vi "Element Init.vi"(7 "VolatusAPI":refnum<class "VolatusAPI.lvclass">, 8 "error in (no error)":errorcluster, 10 "JSON":string, 11 "HtmlButtonControl in":refnum<class "HttpButtonControl.lvclass">) -> (0 "error out":errorcluster, 3 "HtmlButtonControl out":refnum<class "HttpButtonControl.lvclass">)   [LabVIEW 2020, in "VolatusGUIElements.lvlib" / "HttpButtonControl.lvclass"]
uses:
  HttpButtonControl.lvclass
  C:/dev/lv20CE/relink/lv-volatus/VolatusGUI/GUI Element/GUI Element.lvclass
  Volatus/VolatusAPI/VolatusAPI.lvclass
  JSON.ctl
  Method.ctl
  VolatusGUI/GUI Element/GUI Element.lvclass/GUI Element.ctl
  HttpButtonControl.lvclass/HttpButtonControl.ctl
  af0a34e3-17dd-43c9-97df-e95964bc46e3.vi
  <vilib>/JDP Science/JSONtext/JSON text to Variant.vi
  <vilib>/JDP Science/JSONtext/LVClass Serializer/JSONtext LVClass Serializer.lvclass
  VolatusGUI/GUI Element/GUI Element.lvclass
  C:/dev/lv20CE/relink/lv-volatus/VolatusGUIElements/HttpButtonControl/HttpButtonControl.lvclass
  C:/dev/lv20CE/relink/lv-volatus/VolatusGUI/OnValueChangeHandler/OnValueChangeHandler.lvclass
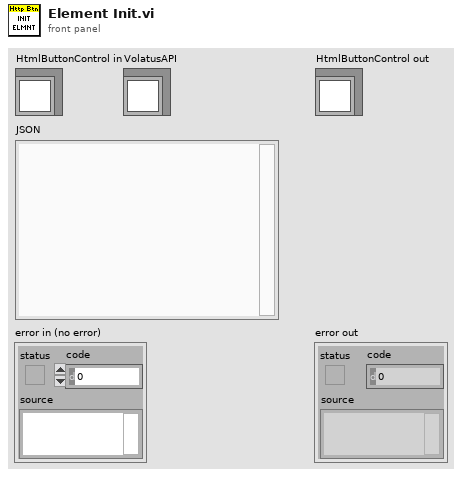
[diagram p1: front panel]
types:
  T1 = typedef "VolatusGUIElements.lvlib/HttpButtonControl.lvclass/Method.ctl" = enum16{"Get", "Post"}
  T2 = typedef "VolatusGUIElements.lvlib/HttpButtonControl.lvclass/JSON.ctl" = cluster{"Method":string, "URL":string, "Toggle":bool, "True":string, "False":string}
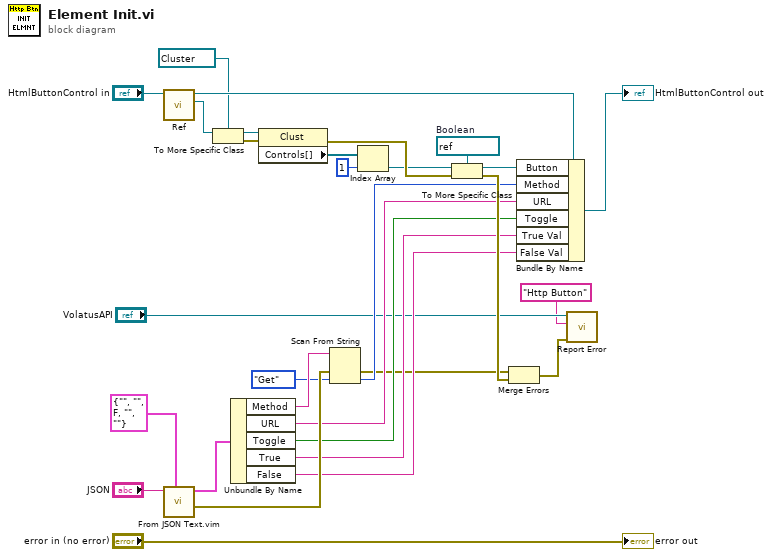
[diagram p0: block diagram]
diagram:
  w17 = refnum<vi> refnum  # Boolean
  n1 = call "Ref.vi"("GUI Element in"="HtmlButtonControl in") -> ("Ref"=w13:refnum<vi>, "GUI Element out"=w21:refnum<class "HttpButtonControl.lvclass">)  [unwired: 9 in]
  n2 = call "From JSON Text.vim"("Data Type and Default Value"=T2 {"Method"="", "URL"="", "Toggle"=FALSE, "True"="", "False"=""} ("JSON"), "JSON"="JSON") -> ("error out"=w22:errorcluster, "Data out"=w24:T2)  [unwired: 8 in]
  n3 = To More Specific Class(target class=refnum<vi> refnum ("specific class reference"), reference=w13) -> (specific class reference=w19:refnum<vi>, error out=w18:errorcluster)  [unwired: 1 in]
  n4 = Unbundle By Name(w24) -> ("Method"=w23:string, "URL"=w10:string, "Toggle"=w9:bool, "True"=w8:string, "False"=w7:string)
  n5 = property class="Clust"(reference=w19, error in=w18) -> (error out=w29:errorcluster, "Controls[]"=w16:refnum<vi>[])  [unwired: 1 out]
  n6 = Scan From String(input string=w23, error in=w22, default 1=Method."Get" ("Method")) -> (error out=w4:errorcluster, output 1=w5:T1)  [unwired: 2 in, 2 out]
  n7 = Index Array(array=w16, index=1) -> (element=w14:refnum<vi>)
  n8 = To More Specific Class(target class=w17, reference=w14, error in=w29) -> (specific class reference=w11:refnum<vi>, error out=w30:errorcluster)
  n9 = Merge Errors(w4, w30) -> (w2:errorcluster)
  n10 = Bundle By Name(cluster=w21, "Button"=w11, "Method"=w5, "URL"=w10, "Toggle"=w9, "True Val"=w8, "False Val"=w7) -> (→"HtmlButtonControl out":refnum<class "HttpButtonControl.lvclass">)
  n11 = call "Report Error.vi"("error in (no error)"=w2, "Context"="Http Button", "VolatusAPI in"="VolatusAPI") -> ()  [unwired: 7 in, 2 out]
  "error out" <- "error in (no error)"
